vi "SLL DE csv File Driver.vi"(7 "Datalog Driver Cases":T2, 8 "error in(no error)":errorcluster, 9 "Data In":sgl[][](array[numeric]), 10 "Time Array":timestamp[](array[timestamp]), 11 "Datalog path (use dialog)":path=path "C:/Documents and Settings/Administrator/Desktop/BXK273640_jesus800.jpg") -> (0 "error out":errorcluster, 1 "Time List":string[](array[string]), 2 "size (in bytes)":i64, 3 "Data Out":dbl[][](array[numeric]), 5 "Channel Names":string[](array[string]))   [LabVIEW 2009]
uses:
  Controls/SLL DE Virtual Chart Datalog Driver Options.ctl
  DAQ Engine/Controls/SLL DE List of Analog Inputs.ctl
panel:
  in  "List of Analog Inputs":T1
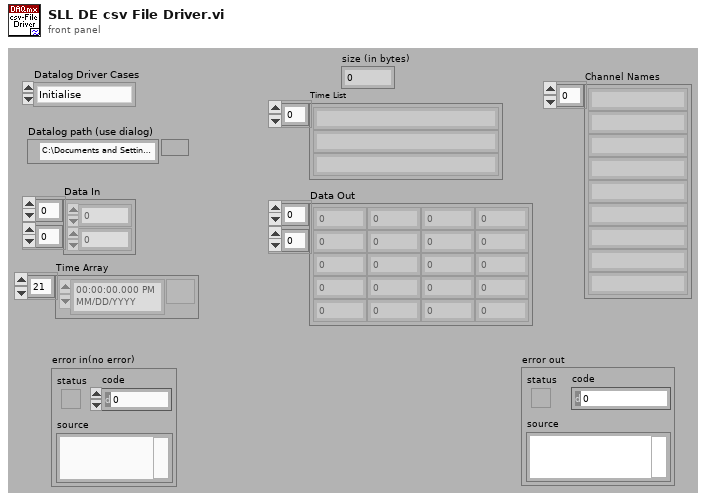
[diagram p1: front panel]
types:
  T1 = typedef "SLL DE List of Analog Inputs.ctl" = enum16{"None"}
  T2 = typedef "SLL DE Virtual Chart Datalog Driver Options.ctl" = enum16{"Initialise", "Write Headings", "Write", "Check File Size", "Read", "Clear"}
  T3 = enum16{"open", "replace", "create", "open or create", "replace or create", "replace or create with confirmation"}
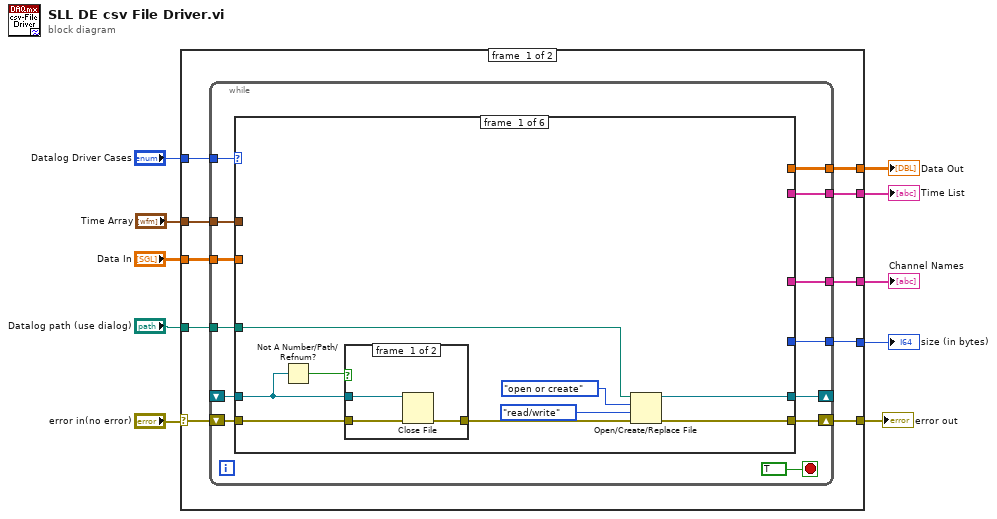
[diagram p0: block diagram]
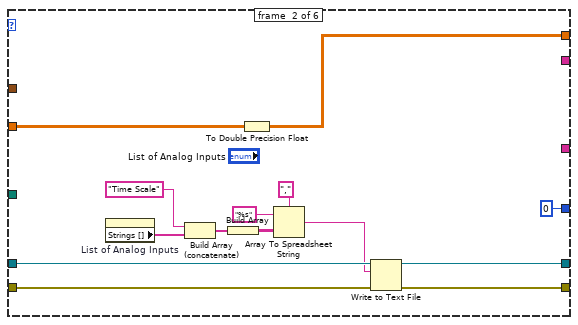
[diagram p3: hidden frame]
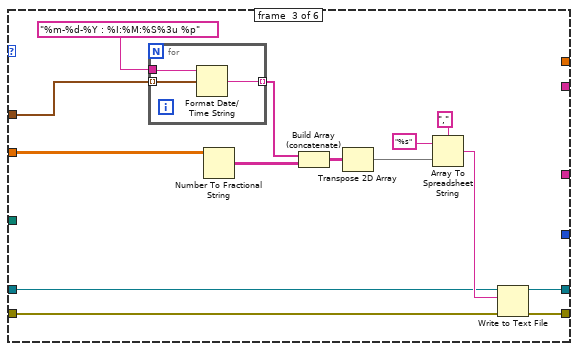
[diagram p4: hidden frame]
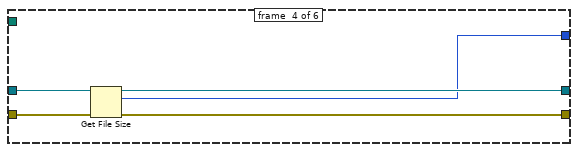
[diagram p5: hidden frame]
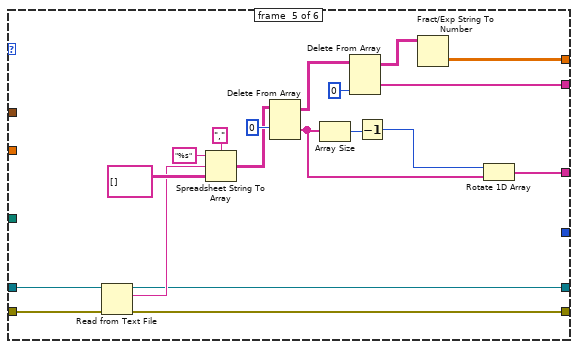
[diagram p6: hidden frame]
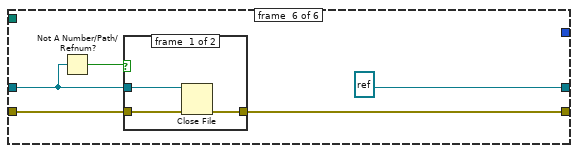
[diagram p7: hidden frame]
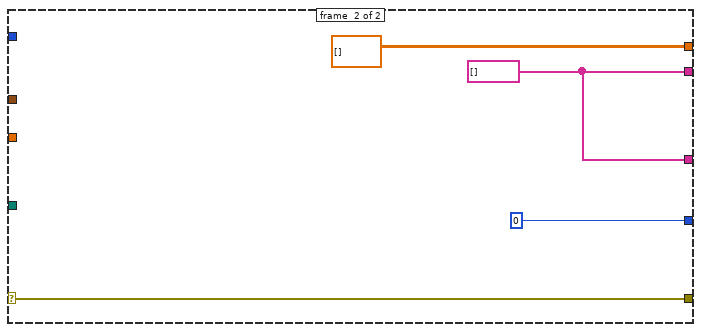
[diagram p9: hidden frame]
diagram:
  n1 = case shown="No Error" "error in(no error)" {
    selector: "error in(no error)" -> [w19 w114]
    tunnel: "Datalog Driver Cases" -> [w20 _]
    tunnel: "Data In" -> [w18 _]
    tunnel: [w17 w114] -> w8
    tunnel: "Datalog path (use dialog)" -> [w16 _]
    tunnel: [w15 dbl[][] []] -> w6
    tunnel: "Time Array" -> [w14 _]
    tunnel: [w13 i64 0 ("size (in bytes)")] -> w3
    tunnel: [w12 w112] -> w2
    tunnel: [w11 w112] -> w1
    frame #0 {
      n2 = while {
        tunnel: w20 -> [w32]
        tunnel: w18 -> [w30]
        shift-right: [w29] -> w17
        shift-left: w19 -> [w31]
        tunnel: w16 -> [w28]
        tunnel: [w27] -> w15
        shift-right: [w26] -> _
        shift-left: _ -> [w25]
        tunnel: w14 -> [w24]
        tunnel: [w23] -> w13
        tunnel: [w22] -> w12
        tunnel: [w21] -> w11
        stop <- TRUE stop-if-true
        n3 = case shown="\"Write Headings\"" w32 {
          tunnel: w31 -> [w38 w57 w70 w82 w90 w105]
          tunnel: w30 -> [_ w60 w62 _ _ _]
          tunnel: [w35 w56 w69 w80 w88 w104] -> w29
          tunnel: w28 -> [w34 _ _ _ _ _]
          tunnel: [_ w59 _ _ w85 _] -> w27
          tunnel: [w36 w55 w71 w79 w86 refnum<file> refnum ("refnum out")] -> w26
          tunnel: w25 -> [w37 w54 w72 w81 w89 w103]
          tunnel: w24 -> [_ _ w66 _ _ _]
          tunnel: [_ i64 0 ("size (in bytes)") _ w78 _ _] -> w23
          tunnel: [_ _ _ _ w84 _] -> w22
          tunnel: [_ _ _ _ w83 _] -> w21
          frame #0 {
            n4 = Not A Number/Path/Refnum?(number/path/refnum=w37) -> (NaN/Path/Refnum?=w40:bool)
            n5 = case shown="False" w40 {
              tunnel: w37 -> [w45 _]
              tunnel: w38 -> [w44 w46]
              tunnel: [w43 w46] -> w39
              frame #0 {
                n6 = Close File(refnum=w45, error in=w44) -> (error out=w43:errorcluster)  [unwired: 1 out]
              }
              frame #1 {
              }
            }
            n7 = Open/Create/Replace File(file path (use dialog)=w34, error in=w39, operation (0:open)=T3."open or create", access (0:read/write)=enum16{"read/write", "read-only", "write-only"}."read/write") -> (refnum out=w36:refnum<file>, error out=w35:errorcluster)  [unwired: 2 in, 1 out]
          }
          frame #1 {
            n8 = property on="List of Analog Inputs" class="Enum (strict)"() -> ("Strings []"=w50:string[])  [unwired: 2 in, 2 out]
            n9 = Build Array (concatenate)("Time Scale", w50) -> (w49:string[])
            n10 = Build Array(w49) -> (w51:string[][])
            n11 = To Double Precision Float(number=w60) -> (double precision float=w59:dbl[][])
            n12 = Array To Spreadsheet String(delimiter (Tab)=",", array=w51, 3:"%s" ("format string")) -> (spreadsheet string=w47:string)
            n13 = Write to Text File(file (use dialog)=w54, text=w47, error in=w57) -> (refnum out=w55:refnum<file>, error out=w56:errorcluster)  [unwired: 1 in, 1 out]
          }
          frame #2 {
            n14 = for {
              tunnel: w66 -> [w77] mode=indexing
              tunnel: [w76] -> w63 mode=indexing
              tunnel: "%m-%d-%Y : %I:%M:%S%3u %p" ("time format string (%c)") -> [w75]
              n15 = Format Date/Time String(time format string (%c)=w75, seconds (now)=w77) -> (date/time string=w76:string)  [unwired: 1 in]
            }
            n16 = Number To Fractional String(number=w62) -> (F-format string=w64:string[][])  [unwired: 3 in]
            n17 = Build Array (concatenate)(w63, w64) -> (w65:string[][])
            n18 = Transpose 2D Array(2D array=w65) -> (transposed array=w67:string[][])
            n19 = Array To Spreadsheet String(delimiter (Tab)=",", array=w67, 3:"%s" ("format string")) -> (spreadsheet string=w73:string)
            n20 = Write to Text File(file (use dialog)=w72, text=w73, error in=w70) -> (refnum out=w71:refnum<file>, error out=w69:errorcluster)  [unwired: 1 in, 1 out]
          }
          frame #3 {
            n21 = Get File Size(file=w81, error in=w82) -> (refnum out=w79:refnum<file>, size (in bytes)=w78:i64, 0:w80:errorcluster)
          }
          frame #4 {
            n22 = Read from Text File(file (use dialog)=w89, error in=w90) -> (refnum out=w86:refnum<file>, text=w87:string, error out=w88:errorcluster)  [unwired: 2 in, 1 out]
            n23 = Spreadsheet String To Array(delimiter (Tab)=",", format string="%s", spreadsheet string=w87, array type (2D Dbl)=string[][] []) -> (array=w94:string[][])
            n24 = Delete From Array(array=w94, index (row)=0) -> (deleted portion=w99:string[], array with subset deleted=w95:string[][])  [unwired: 2 in]
            n25 = Array Size(array=w99) -> (size(s)=w100:i32)
            n26 = Delete From Array(array=w95, index (col)=0 ("disabled index (col)")) -> (deleted portion=w84:string[], array with subset deleted=w98:string[][])  [unwired: 2 in]
            n27 = Decrement(x=w100) -> (x-1=w101:i32)
            n28 = Fract/Exp String To Number(string=w98) -> (number=w85:dbl[][])  [unwired: 3 in, 1 out]
            n29 = Rotate 1D Array(1:w99, 2:w101) -> (0:w83:string[])
          }
          frame #5 {
            n30 = Not A Number/Path/Refnum?(number/path/refnum=w103) -> (NaN/Path/Refnum?=w102:bool)
            n31 = case shown="False" w102 {
              tunnel: w103 -> [w109 _]
              tunnel: w105 -> [w108 w110]
              tunnel: [w107 w110] -> w104
              frame #0 {
                n32 = Close File(refnum=w109, error in=w108) -> (error out=w107:errorcluster)  [unwired: 1 out]
              }
              frame #1 {
              }
            }
          }
        }
      }
    }
    frame #1 {
      w112 = string[] []
    }
  }
  "error out" <- w8
  "Data Out" <- w6
  "size (in bytes)" <- w3
  "Time List" <- w2
  "Channel Names" <- w1
